vi "PDC_GetShadingModeList.vi"(8 "error in (no error)":errorcluster, 10 "ChildNo":u32, 11 "DeviceNo":u32) -> (0 "error out":errorcluster, 1 "List":u32[](array[numeric]), 2 "Size":u32, 3 "ReturnValue":u32, 4 "ErrorCode":u32)   [LabVIEW 2015]
doc: "This VI retrieves the list of shading modes that can be set in the specified child device."
uses:
  sub/global.vi
  PDCLIB.dll
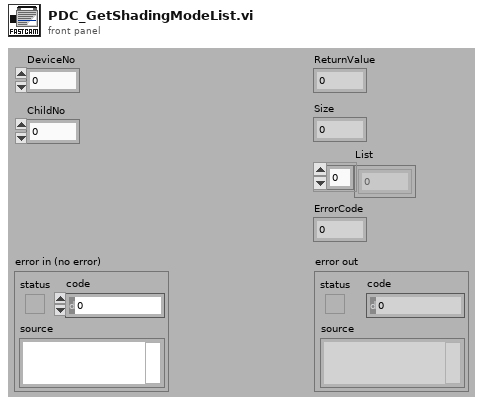
[diagram p1: front panel]
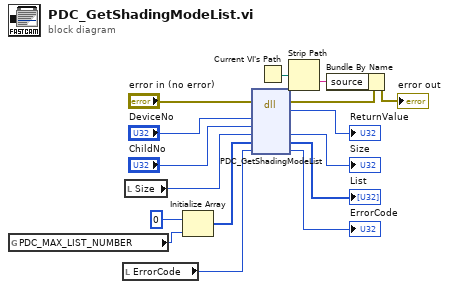
[diagram p0: block diagram]
diagram:
  n1 = global read "global.vi" "PDC_MAX_LIST_NUMBER"() -> (w9:i32)
  n2 = local read "ErrorCode"() -> (w13:u32)
  n3 = local read "Size"() -> (w10:u32)
  n4 = Initialize Array(u32 0, w9) -> (w8:u32[])
  n5 = dll-call lib="PDCLIB.dll" fn="PDC_GetShadingModeList"(error in="error in (no error)", "nDeviceNo"="DeviceNo", "nChildNo"="ChildNo", "pSize"=w10, "pList"=w8, "pErrorCode"=w13) -> (error out=w2:errorcluster, "return type"=→"ReturnValue":u32, "pSize"=→"Size":u32, "pList"=→"List":u32[], "pErrorCode"=→"ErrorCode":u32)  [unwired: 4 in, 1 out]
  n6 = Current VI's Path() -> (path=w3:path)
  n7 = Strip Path(path=w3) -> (name=w4:string)  [unwired: 1 out]
  n8 = Bundle By Name(cluster=w2, "source"=w4) -> (→"error out":errorcluster)
